vi "DelayScan.NPoints.vi"(9 "Mono":T1={"offset (cm-1)"=200.0, "step (cm-1)"=2.0, "Counter"=146.4557703573521, "Scanstep/monostep"=20, "Status"={"Moving"=FALSE, "Home"=FALSE, "Hi"=FALSE, "Low"=FALSE}, "nm"=585.8230814294084, "Mono port"="COM7"} {"nm" format="%.3f"; "Counter" format="%.2g"; "step (cm-1)" format="%.1f"}, 10 "DyeLaser In":T3={"Scan.Start (cm-1)"=15000.0, "Scan.Stop (cm-1)"=15050.0, "Scan.step (cm-1)"=0.2, "dye laser port"="", "Laser"=enum."Syrah", "NPoints"=251, "CurrentStep"=75, "Current.cm-1"=15015.0} {"Current.cm-1" format="%.2f"}, 11 "Camera":T2={"Gate.Delay"=0, "Delay.Step"=0, "Gate.Duration"=150000, "#Accum"=10, "SetpointTemp"=-30, "Last Temp"=6, "Current Temp"=4}) -> (0 "Final.Gate.Delay":u64, 1 "Mono out":T1, 2 "DyeLaser out":T3={"Scan.Start (cm-1)"=15000.0, "Scan.Stop (cm-1)"=15050.0, "Scan.step (cm-1)"=0.2, "dye laser port"="", "Laser"=enum."Syrah", "NPoints"=251, "CurrentStep"=75, "Current.cm-1"=15015.0} {"Current.cm-1" format="%.2f"}, 3 "Camera out":T2)   [LabVIEW 2022 SP3]
panel:
  # "ns"
  # "ns"
  # "ns"
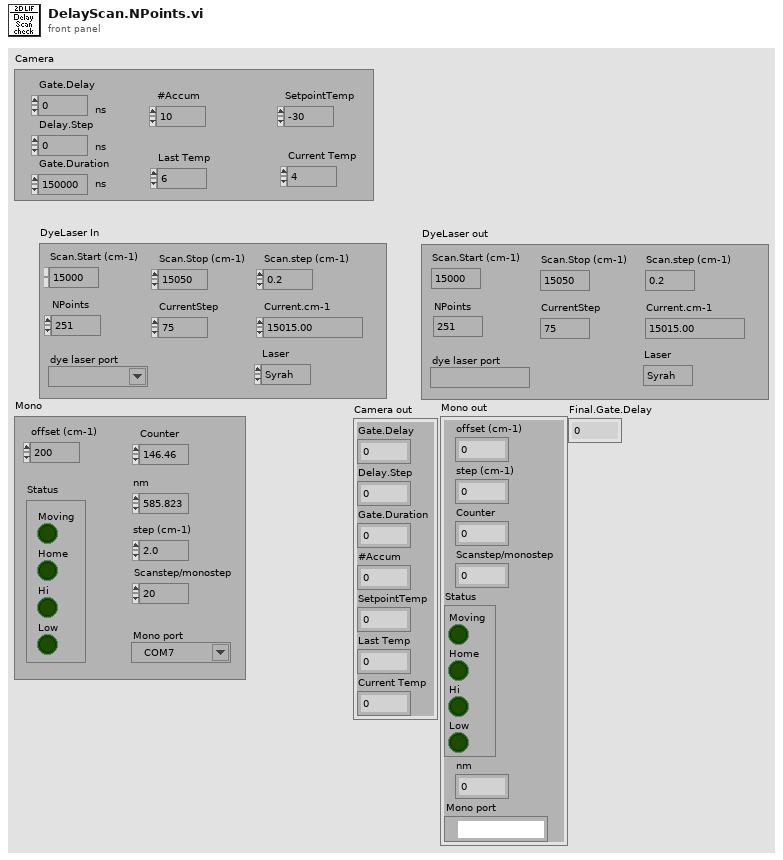
[diagram p1: front panel]
types:
  T1 = cluster{"offset (cm-1)":dbl, "step (cm-1)":dbl, "Counter":dbl, "Scanstep/monostep":i32, "Status":cluster{"Moving":bool, "Home":bool, "Hi":bool, "Low":bool}, "nm":dbl, "Mono port":refnum<visa-resource-name>}
  T2 = cluster{"Gate.Delay":u64, "Delay.Step":u64, "Gate.Duration":u64, "#Accum":i32, "SetpointTemp":i32, "Last Temp":i32, "Current Temp":i32}
  T3 = cluster{"Scan.Start (cm-1)":dbl, "Scan.Stop (cm-1)":dbl, "Scan.step (cm-1)":dbl, "dye laser port":refnum<visa-resource-name>, "Laser":enum16{"Syrah", "Hyperdye"}, "NPoints":i32, "CurrentStep":i32, "Current.cm-1":dbl}
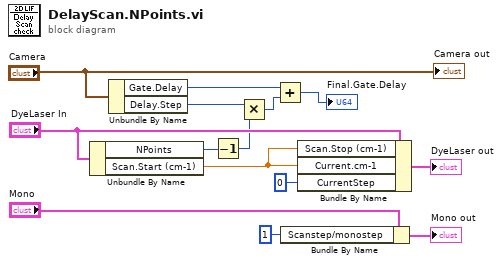
[diagram p0: block diagram]
diagram:
  n1 = Unbundle By Name("DyeLaser In") -> ("NPoints"=w6:i32, "Scan.Start (cm-1)"=w12:dbl)
  n2 = Unbundle By Name("Camera") -> ("Gate.Delay"=w3:u64, "Delay.Step"=w2:u64)
  n3 = Decrement(x=w6) -> (x-1=w5:i32)
  n4 = Multiply(x=w2, y=w5) -> (x*y=w4:u64)
  n5 = Add(x=w3, y=w4) -> (x+y=→"Final.Gate.Delay":u64)
  n6 = Bundle By Name(cluster="Mono", "Scanstep/monostep"=1) -> (→"Mono out":T1)
  n7 = Bundle By Name(cluster="DyeLaser In", "Scan.Stop (cm-1)"=w12, "Current.cm-1"=w12, "CurrentStep"=0) -> (→"DyeLaser out":T3)
  "Camera out" <- "Camera"
